vi "像素操作之边框和文字.vi"() -> ()   [LabVIEW 2018]
uses:
  <vilib>/vision/NI_Vision_Development_Module.lvlib
panel:
  out "Image 2":T1(plugin-control)
  out "error out":errorcluster
  out "Image":T1(plugin-control)
  in  "路径":path
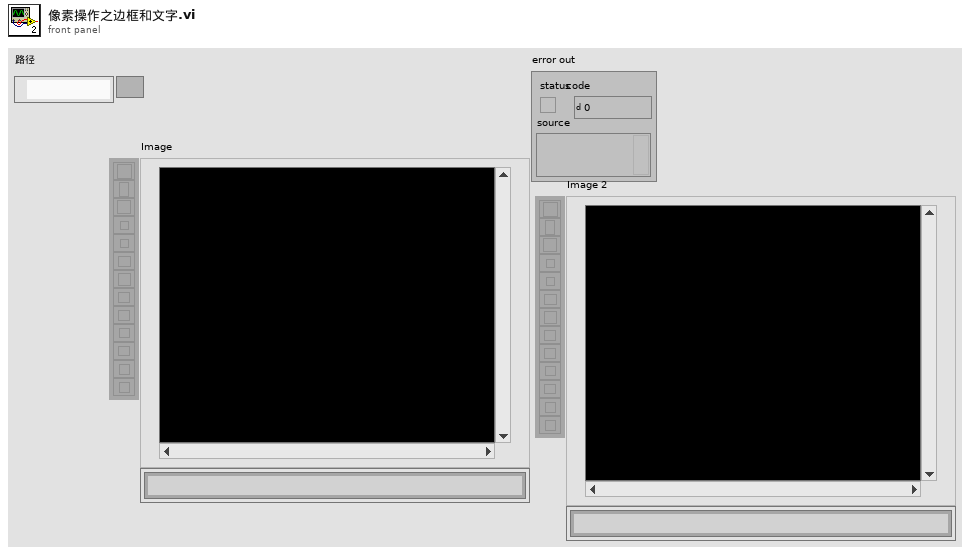
[diagram p1: front panel]
types:
  T1 = typedef "IMAQ Image.ctl" = refnum<image>
  T2 = cluster{"Desired Font (Application)":enum16{"User-specified Font", "Application Font", "System Font", "Dialog Font"}, "[User-specified Font]":cluster{"Font Name":string, "Size":i16, "Strikeout?":bool, "Italic?":bool, "Underline?":bool, "Outline?":bool, "Shadow?":bool, "Bold?":bool, "Rotation Angle":dbl}, "Horizontal Alignment":i16, "Vertical Alignment":i16}
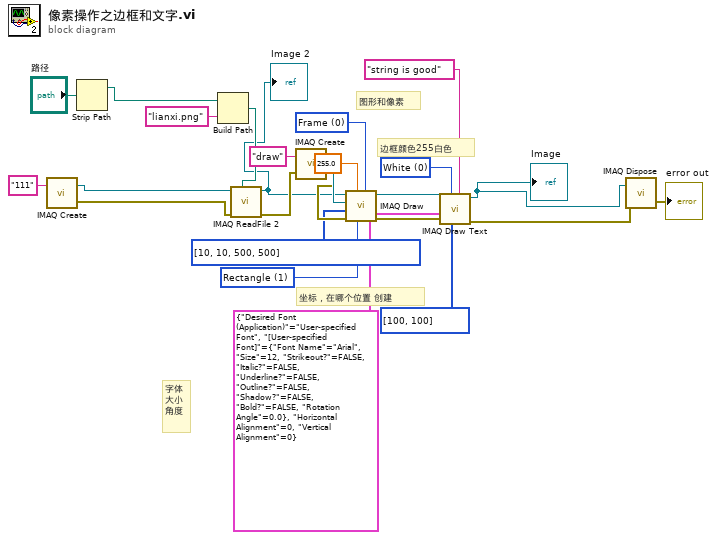
[diagram p0: block diagram]
diagram:
  w6 = 0 items=["White", "Black", "Inverted", "Black on White", "White on Black"] ("Color")
  w11 = u16 1 items=["Line", "Rectangle", "Oval"] ("Shape to draw")
  w12 = u16 0 items=["Frame", "Paint", "Invert Frame", "Invert Paint"] ("Draw Mode")
  # "字体\n大小\n角度"
  # "图形和像素"
  # "边框颜色255白色"
  # "坐标，在哪个位置 创建"
  n1 = call "IMAQ Create"("Image Name"="111") -> ("New Image"=w21:T1, "error out"=w20:errorcluster)  [unwired: 4 in]
  n2 = Strip Path(path="路径") -> (stripped path=w24:path)  [unwired: 1 out]
  n3 = Build Path(base path=w24, name or relative path="lianxi.png" ("名称或相对路径")) -> (appended path=w19:path)
  n4 = call "IMAQ ReadFile 2"("File Path"=w19, "error in (no error)"=w20, "Image"=w21) -> ("error out"=w16:errorcluster, "Image Out"=w3:T1)  [unwired: 4 in, 3 out]
  "Image 2" <- w3
  n5 = call "IMAQ Create"("Image Name"="draw", "error in (no error)"=w16) -> ("New Image"=w17:T1, "error out"=w15:errorcluster)  [unwired: 3 in]
  n6 = call "IMAQ Draw"("Draw Mode"=w12, "Shape to draw"=w11, "Pixel Color"=sgl 255.0, "error in (no error)"=w15, "Coordinates"=i32[] [10, 10, 500, 500], "Image Dst"=w17, "Image Src"=w3) -> ("error out"=w1:errorcluster, "Image Dst Out"=w2:T1)  [unwired: 3 in]
  n7 = call "IMAQ Draw Text"("String"="string is good", "Insertion Point"=i32[] [100, 100], "Color"=w6, "error in (no error)"=w1, "Font, Size & Style"=T2 {"Desired Font (Application)"=enum."User-specified Font", "[User-specified Font]"={"Font Name"="Arial", "Size"=12, "Strikeout?"=FALSE, "Italic?"=FALSE, "Underline?"=FALSE, "Outline?"=FALSE, "Shadow?"=FALSE, "Bold?"=FALSE, "Rotation Angle"=0.0}, "Horizontal Alignment"=0, "Vertical Alignment"=0}, "Image Src"=w2) -> ("error out"=w7:errorcluster, "Image Dst Out"=w8:T1)  [unwired: 2 in, 2 out]
  "Image" <- w8
  n8 = call "IMAQ Dispose"("Image"=w8, "error in (no error)"=w7) -> ("error out"=→"error out":errorcluster)  [unwired: 4 in]
